vi "Server_GET.vi"(8 "error in":errorcluster, 11 "lia rt in":refnum<class "Lock-In Amplifier Example RT.lvclass">) -> (0 "error out":errorcluster, 2 "server":refnum<class "RT FlexRIO Server TCP.lvclass">, 3 "lia rt out":refnum<class "Lock-In Amplifier Example RT.lvclass">)   [LabVIEW 2017, in "Lock-In Amplifier Example RT.lvclass"]
uses:
  Lock-In Amplifier Example RT.lvclass
  server/RT FlexRIO Server TCP.lvclass
  Lock-In Amplifier Example RT.lvclass/Lock-In Amplifier Example RT.ctl
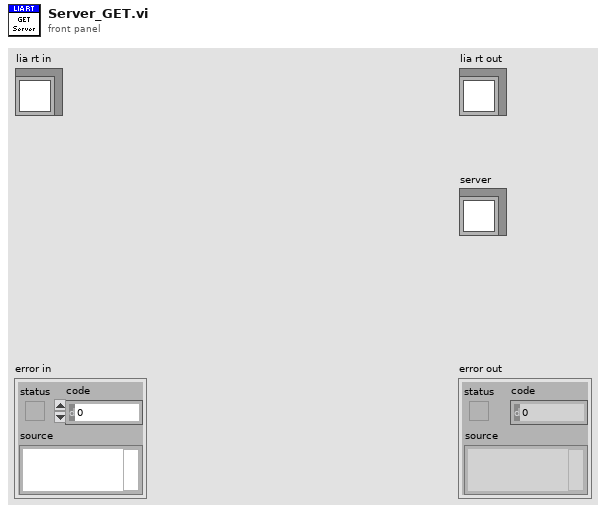
[diagram p1: front panel]
types:
  T1 = typedef "Lock-In Amplifier Example RT.lvclass/session data.ctl" = cluster{"server":refnum<class "RT FlexRIO Server TCP.lvclass">, "fpga interface":refnum<class "LIA Host Interface FPGA.lvclass">}
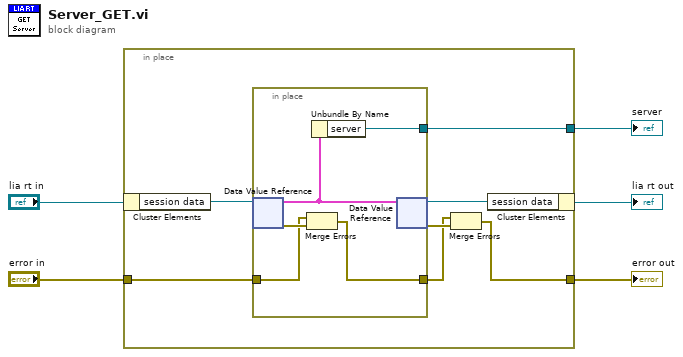
[diagram p0: block diagram]
diagram:
  n1 = in-place {
    in-place-border: [w10] -> w1
    in-place-border: "error in" -> [w9]
    in-place-border: [w6] -> w2
    n2 = in-place-cluster #1("lia rt in") -> ("session data"=w12:refnum<data-value>)
    n3 = in-place {
      in-place-border: [w16] -> w10
      in-place-border: w9 -> [w14]
      in-place-border: [w13] -> w7
      n4 = in-place-dvr #2(w12) -> (w17:T1, w15:errorcluster)
      n5 = Merge Errors(w14, w15) -> (w13:errorcluster)
      n6 = Unbundle By Name(w17) -> ("server"=w16:refnum<class "RT FlexRIO Server TCP.lvclass">)
      n7 = in-place-dvr #2(w17) -> (w11:refnum<data-value>, w8:errorcluster)
    }
    n8 = Merge Errors(w7, w8) -> (w6:errorcluster)
    n9 = in-place-cluster #1("session data"=w11) -> (→"lia rt out":refnum<class "Lock-In Amplifier Example RT.lvclass">)
  }
  "error out" <- w2
  "server" <- w1
